vi "MaxArray.vi"(0 "Array":fxp<+/-,32,16>[](array[numeric])) -> (1 "Max":fxp<+/-,32,16> format="%.21g", 2 "Max Index":i32, 3 "Min":fxp<+/-,32,16> format="%.21g", 4 "Min Index":i32)   [LabVIEW 2015]
uses:
  <vilib>/rvi/Emulation/niFpgaGetClockAttributes.vi
  <vilib>/rvi/Emulation/niFpgaSctlEmulationGetInTimedLoop.vi
  <vilib>/rvi/Emulation/niFpgaEmulationReportErrorSimple.vi
  <vilib>/rvi/Emulation/niFpgaCriticalErrorInLSC.vi
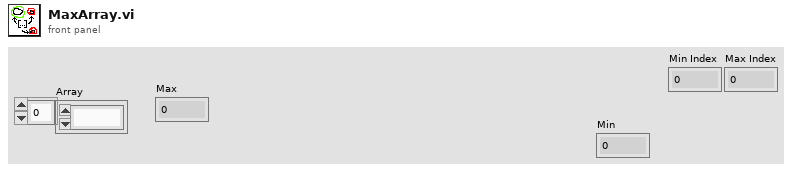
[diagram p1: front panel]
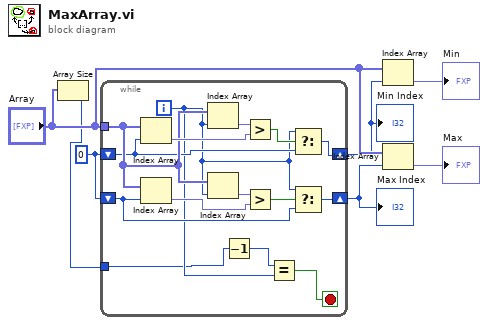
[diagram p0: block diagram]
diagram:
  w5 = u16 0
  n1 = Array Size(array="Array") -> (size(s)=w1:i32)
  n2 = while {
    tunnel: "Array" -> [w14]
    shift-right: [w18] -> w6
    shift-left: w5 -> [w19]
    shift-right: [w13] -> w3
    shift-left: w5 -> [w12]
    tunnel: w1 -> [w9]
    i -> [w10]
    stop <- w11 stop-if-true
    n3 = Index Array(array=w14, index=w12) -> (element=w16:fxp<+/-,32,16>)
    n4 = Index Array(array=w14, index=w19) -> (element=w21:fxp<+/-,32,16>)
    n5 = Index Array(array=w14, index=w10) -> (element=w17:fxp<+/-,32,16>)
    n6 = Index Array(array=w14, index=w10) -> (element=w22:fxp<+/-,32,16>)
    n7 = Decrement(x=w9) -> (x-1=w8:i32)
    n8 = Greater?(x=w17, y=w16) -> (0:w15:bool)
    n9 = Greater?(x=w22, y=w21) -> (0:w20:bool)
    n10 = Equal?(x=w8, y=w10) -> (x = y?=w11:bool)
    n11 = Select(t=w10, s=w15, f=w12) -> (s? t:f=w13:i32)
    n12 = Select(t=w10, s=w20, f=w19) -> (s? t:f=w18:i32)
  }
  "Min Index" <- w3
  "Max Index" <- w6
  n13 = Index Array(array="Array", index=w3) -> (element=→"Min":fxp<+/-,32,16>)
  n14 = Index Array(array="Array", index=w6) -> (element=→"Max":fxp<+/-,32,16>)
